vi "Threshold (Otsu).vi"(4 "Max Value (Default: 255)":u8=255, 6 "Invert? (Default: False)":bool, 8 "error in (no error)":errorcluster, 10 "Otsu Threshold Result":T1, 11 "Greyscale Image-Source":T1) -> (0 "error out":errorcluster, 3 "Otsu Threshold Result (duplicate)":T1)   [LabVIEW 2020, in "g_ar_toolkit.image.lvlib"]
uses:
  g_ar_toolkit.image.lvlib
  Greyscale Image.ctl
  ThresholdTypes.ctl
  g_ar_toolkit.common/Module Path.vi
  <vilib>/Utility/error.llb/Error Cluster From Error Code.vi
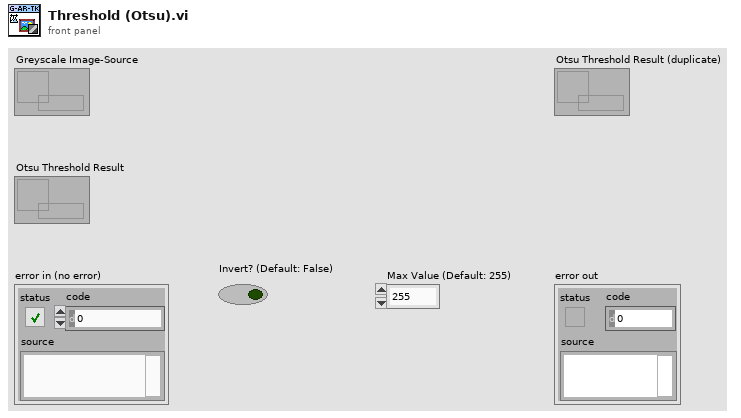
[diagram p1: front panel]
types:
  T1 = typedef "g_ar_toolkit.image.lvlib/Greyscale Image.ctl" = refnum<data-value>
  T2 = typedef "g_ar_toolkit.image.lvlib/ThresholdTypes.ctl" = enum8{"THRESH_BINARY", "THRESH_BINARY_INV", "THRESH_TRUNC", "THRESH_TOZERO", "THRESH_TOZERO_INV", "THRESH_MASK", "THRESH_OTSU", "THRESH_TRIANGLE"}
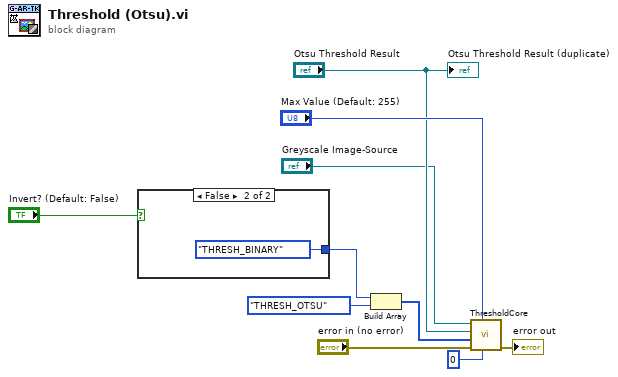
[diagram p0: block diagram]
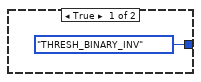
[diagram p2: hidden frame]
diagram:
  n1 = case shown="False" "Invert? (Default: False)" {
    tunnel: [ThresholdTypes."THRESH_BINARY_INV" ("Threshold Types") ThresholdTypes."THRESH_BINARY" ("Threshold Types")] -> w3
    frame True {
    }
    frame False {
    }
  }
  n2 = Build Array(w3, ThresholdTypes."THRESH_OTSU" ("element")) -> (w1:T2[])
  n3 = call "ThresholdCore.vi"("Threshold"=u8 0, "Max Value"="Max Value (Default: 255)", "error in (no error)"="error in (no error)", "Mode"=w1, "Threshold Result"="Otsu Threshold Result", "Greyscale Image-Source"="Greyscale Image-Source") -> ("error out"=→"error out":errorcluster)  [unwired: 5 in]
  "Otsu Threshold Result (duplicate)" <- "Otsu Threshold Result"
